vi "WILT Anti Flood Check.vi"(6 "Disable Flood Check":bool, 7 "Current Station Time (Minutes)":dbl, 8 "Error In":errorcluster, 9 "Enable Start Retry":bool, 10 "Previous Cycle Time (Minutes)":dbl, 11 "Station Drying Time (Min)":dbl) -> (0 "Error Out 2":errorcluster, 3 "Shut Valve Off?":bool)   [LabVIEW 2016]
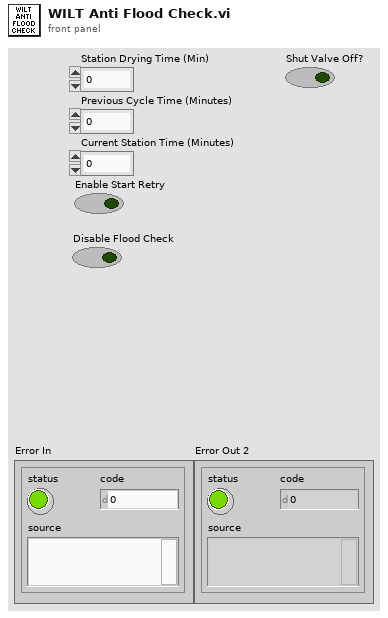
[diagram p1: front panel]
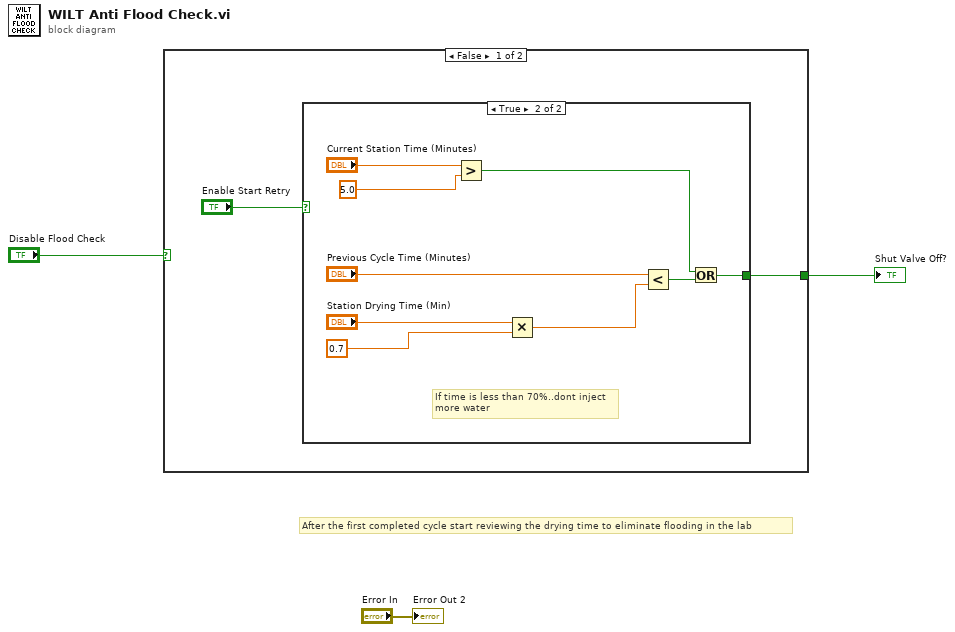
[diagram p0: block diagram]
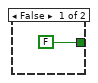
[diagram p2: hidden frame]
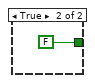
[diagram p3: hidden frame]
diagram:
  # "After the first completed cycle start reviewing the drying time to eliminate flooding in the lab"
  n1 = case shown="False" "Disable Flood Check" {
    tunnel: [w5 FALSE ("Boolean")] -> w3
    frame False {
      n2 = case shown="True" "Enable Start Retry" {
        tunnel: [FALSE w7] -> w5
        frame False {
        }
        frame True {
          # "If time is less than 70%..dont inject\nmore water"
          n3 = Greater?(x="Current Station Time (Minutes)", y=5.0) -> (0:w9:bool)
          n4 = Multiply(x="Station Drying Time (Min)", y=0.7) -> (x*y=w15:dbl)
          n5 = Less?(x="Previous Cycle Time (Minutes)", y=w15) -> (x < y?=w8:bool)
          n6 = Or(x=w9, y=w8) -> (x .or. y?=w7:bool)
        }
      }
    }
    frame True {
    }
  }
  "Shut Valve Off?" <- w3
  "Error Out 2" <- "Error In"
